vi "Get Count.vi"(8 "error in (no error)":errorcluster, 11 "Core Transfers Configuration in":refnum<class "Core Transfers Configuration.lvclass">) -> (0 "error out":errorcluster, 2 "count":i32, 3 "Core Transfers Configuration out":refnum<class "Core Transfers Configuration.lvclass">)   [LabVIEW 2017, in "DSF Core.lvlib" / "Core Transfers Configuration.lvclass"]
uses:
  Core Transfers Configuration.lvclass
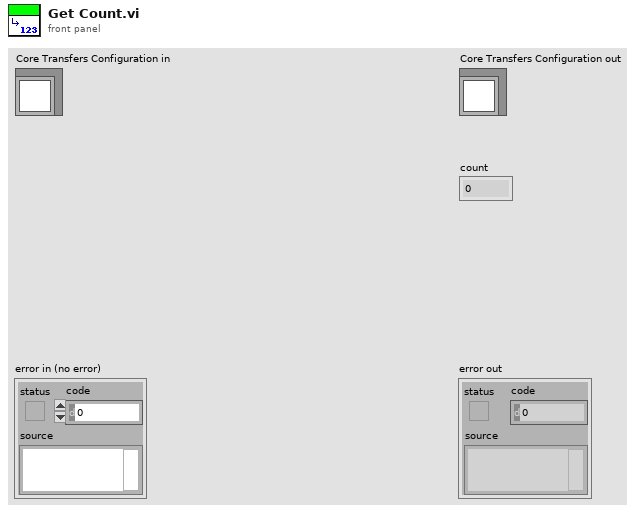
[diagram p1: front panel]
types:
  T1 = typedef "DSF Core.lvlib/Core Transfers Configuration.lvclass/Configuration.ctl" = cluster{"name":string}
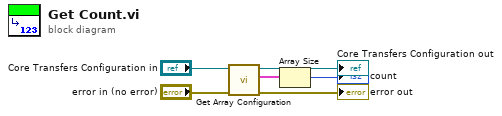
[diagram p0: block diagram]
diagram:
  n1 = call "Get Array Configuration.vi"("error in (no error)"="error in (no error)", "Core Transfers Configuration in"="Core Transfers Configuration in") -> ("error out"=→"error out":errorcluster, "transfer configurations"=w2:T1[], "Core Transfers Configuration out"=→"Core Transfers Configuration out":refnum<class "Core Transfers Configuration.lvclass">)  [unwired: 7 in]
  n2 = Array Size(array=w2) -> (size(s)=→"count":i32)
